vi "basic_Compare Size.vi"(8 "error in (no error)":errorcluster, 10 "size B":i32, 11 "size A":i32) -> (0 "error out":errorcluster)   [LabVIEW 2013, in "NI_EP_Basic.lvlib"]
uses:
  <vilib>/addons/Electrical Power/Basic/NI_EP_Basic.lvlib
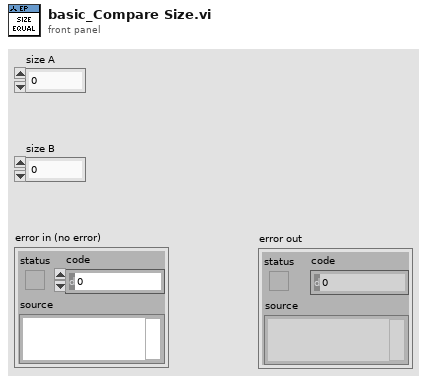
[diagram p1: front panel]
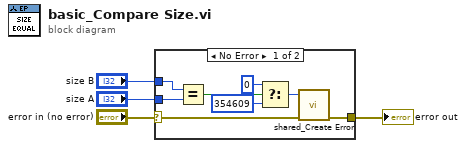
[diagram p0: block diagram]
diagram:
  n1 = case shown="No Error" "error in (no error)" {
    selector: "error in (no error)" -> [w5 w13]
    tunnel: [w8 w13] -> w4
    tunnel: "size A" -> [w7 _]
    tunnel: "size B" -> [w6 _]
    frame No Error {
      n2 = Equal?(x=w6, y=w7) -> (x = y?=w9:bool)
      n3 = Select(t=0, s=w9, f=354609) -> (s? t:f=w12:i32)
      n4 = call <vilib>:"shared_Create Error.vi"("error in (no error)"=w5, "error code (0)"=w12) -> ("error out"=w8:errorcluster)  [unwired: 9 in]
    }
    frame Error {
    }
  }
  "error out" <- w4
